vi "3.vi"() -> ()   [LabVIEW 2015]
panel:
  out "resulting string":string
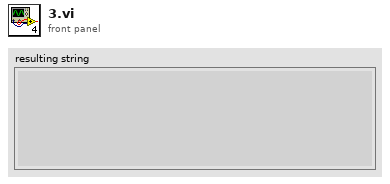
[diagram p1: front panel]
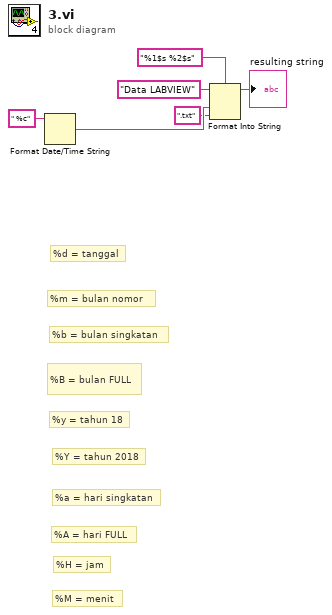
[diagram p0: block diagram]
diagram:
  # "%M = menit"
  # "%H = jam"
  # "%A = hari FULL"
  # "%a = hari singkatan"
  # "%Y = tahun 2018"
  # "%y = tahun 18"
  # "%B = bulan FULL"
  # "%b = bulan singkatan"
  # "%m = bulan nomor"
  # "%d = tanggal"
  n1 = Format Date/Time String(time format string (%c)=" %c") -> (date/time string=w6:string)  [unwired: 2 in]
  n2 = Format Into String(format string="%1$s %2$s", initial string="Data LABVIEW", w6, ".txt" ("input 2")) -> (resulting string=→"resulting string":string)  [unwired: 1 in, 1 out]
